vi "Swap Rows.vi"() -> ()   [LabVIEW 2015]
panel:
  in  "Array out":dbl[](array[numeric])
  in  "Array":dbl[](array[numeric])
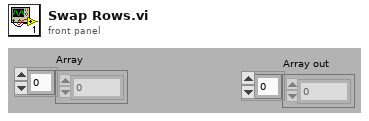
[diagram p1: front panel]
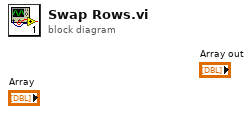
[diagram p0: block diagram]
diagram:
